vi "Oscilloscope Configure.vi"(8 "error in (no error)":errorcluster, 10 "instrument handle":refnum<k15>, 11 "Oscilloscope in":refnum<class "Oscilloscope.lvclass">) -> (0 "error out":errorcluster, 2 "instrument handle out":refnum<k15>, 3 "Oscilloscope out":refnum<class "Oscilloscope.lvclass">)   [LabVIEW 2023, in "HardwareAbstractionLayer_LVOOP.lvlib" / "Oscilloscope.lvclass"]
uses:
  Oscilloscope.lvclass
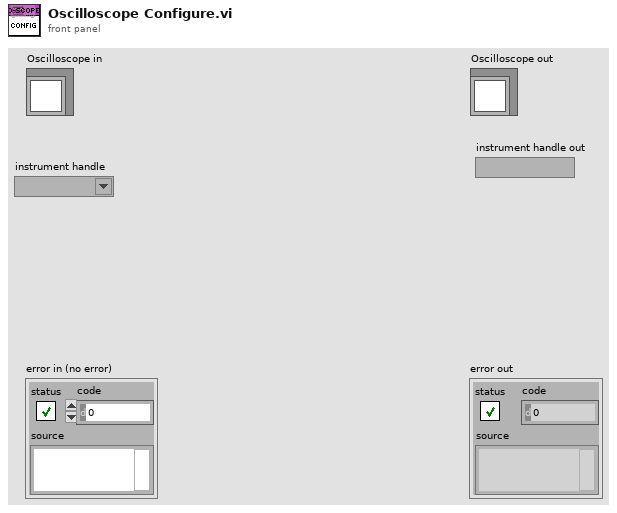
[diagram p1: front panel]
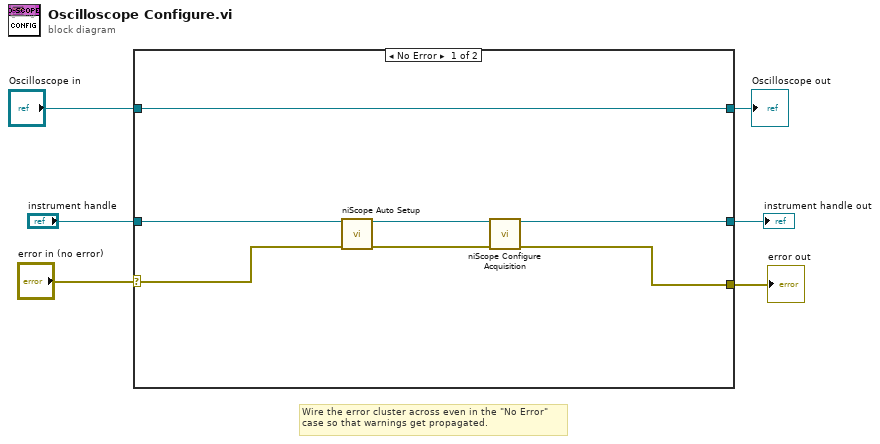
[diagram p0: block diagram]
diagram:
  # "Wire the error cluster across even in the \"No Error\"\ncase so that warnings get propagated."
  n1 = case shown="No Error" "error in (no error)" {
    selector: "error in (no error)" -> [w9 w16]
    tunnel: [w8 w16] -> w5
    tunnel: [w13 w15] -> w3
    tunnel: "Oscilloscope in" -> [w13 w15]
    tunnel: "instrument handle" -> [w10 w14]
    tunnel: [w7 w14] -> w1
    frame No Error {
      n2 = call <instrlib>:"niScope Auto Setup.vi"("instrument handle"=w10, "error in"=w9) -> ("instrument handle out"=w12:refnum<k15>, "error out"=w11:errorcluster)  [unwired: 12 in]
      n3 = call <instrlib>:"niScope Configure Acquisition.vi"("instrument handle"=w12, "error in"=w11) -> ("instrument handle out"=w7:refnum<k15>, "error out"=w8:errorcluster)  [unwired: 12 in]
    }
    frame Error {
    }
  }
  "error out" <- w5
  "Oscilloscope out" <- w3
  "instrument handle out" <- w1
